vi "Process Image for Balls.vi"(0 "Src Image":T1, 1 "Color Mode 2":u16(ring)=2 items=["RGB", "HSL", "HSV", "HSI"], 5 "Image Dst":T1, 9 "Color":T3, 11 "Area Cutoff %":dbl=0.4) -> (4 "Src Image Out":T1, 8 "First Threshold":T1, 10 "Fitted":T1, 15 "Potential":T2(array[cluster]))   [LabVIEW 2015]
doc: "Search image for circular colored particles. A second pass extracts a portion of the image, widens the color range, and fits a circle to the edge of the result."
uses:
  <vilib>/vision/Image Controls.llb/IMAQ Image.ctl
  <vilib>/vision/NI_Vision_Development_Module.lvlib
panel:
  out "Particles":i32
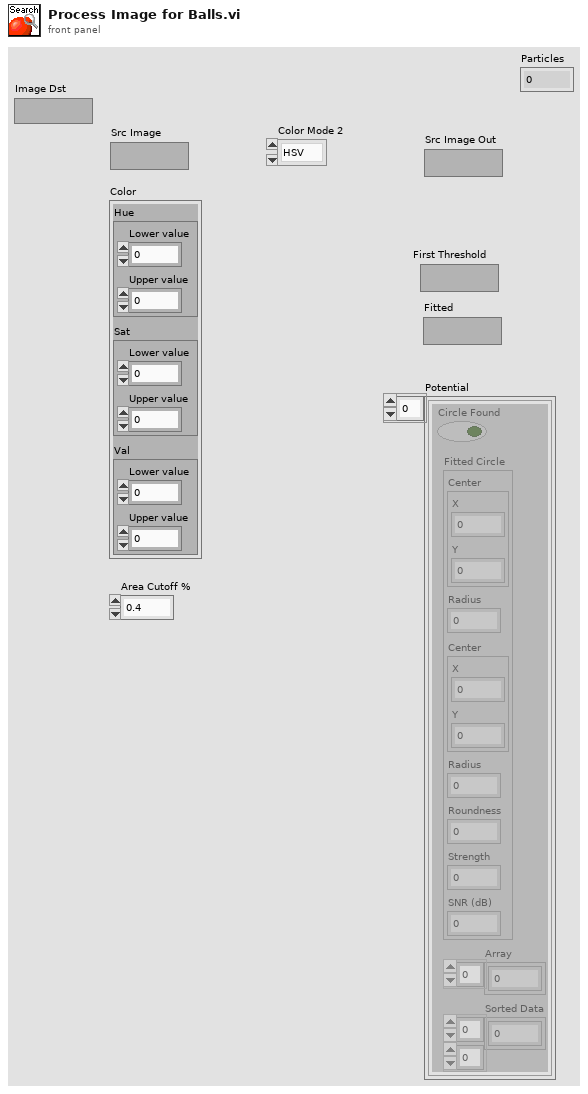
[diagram p1: front panel]
types:
  T1 = typedef "IMAQ Image.ctl" = refnum<image>
  T2 = cluster{"Circle Found":bool, "Fitted Circle":cluster{"Center":cluster{"X":sgl, "Y":sgl}, "Radius":dbl, "Center":cluster{"X":sgl, "Y":sgl}, "Radius":dbl, "Roundness":dbl, "Strength":dbl, "SNR (dB)":dbl}, "Array":dbl[], "Sorted Data":dbl[][]}[]
  T3 = cluster{"Hue ":cluster{"Lower value":i32, "Upper value":i32}, "Sat ":cluster{"Lower value":i32, "Upper value":i32}, "Val ":cluster{"Lower value":i32, "Upper value":i32}}
  T4 = typedef "Particle Parameters" = i32
  T5 = typedef "ROI Descriptor" = cluster{"Global Rectangle":i32[], "Contours":cluster{"ID":enum32{"External", "Internal"}, "Type":u32, "Coordinates":i32[]}[]}
  T6 = cluster{"Circle Found":bool, "Fitted Circle":cluster{"Center":cluster{"X":sgl, "Y":sgl}, "Radius":dbl, "Center":cluster{"X":sgl, "Y":sgl}, "Radius":dbl, "Roundness":dbl, "Strength":dbl, "SNR (dB)":dbl}, "Array":dbl[], "Sorted Data":dbl[][]}
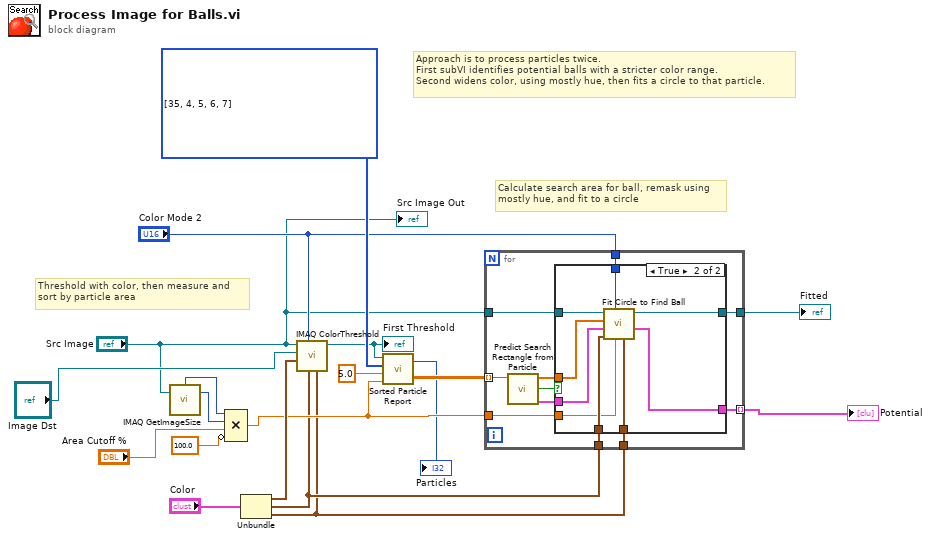
[diagram p0: block diagram]
diagram:
  w18 = T4[] [35, 4, 5, 6, 7] items=["Center of Mass X", "Center of Mass Y", "First Pixel X", "First Pixel Y", "Bounding Rect Left", "Bounding Rect Top", "Bounding Rect Right", "Bounding Rect Bottom", "Max Feret Diameter Start X", "Max Feret Diameter Start Y", "Max Feret Diameter End X", "Max Feret Diameter End Y", "Max Horiz. Segment Length Left", "Max Horiz. Segment Length Right", "Max Horiz. Segment Length Row", "-", "Bounding Rect Width", "Bounding Rect Height", "Bounding Rect Diagonal", "Perimeter", "Convex Hull Perimeter", "Holes' Perimeter", "Max Feret Diameter", "Equivalent Ellipse Major Axis", "Equivalent Ellipse Minor Axis", "Equivalent Ellipse Minor Axis (Feret)", "Equivalent Rect Long Side", "Equivalent Rect Short Side", "Equivalent Rect Diagonal", "Equivalent Rect Short Side (Feret)", "Average Horiz. Segment Length", "Average Vert. Segment Length", "Hydraulic Radius", "Waddel Disk Diameter", "-", "Area", "Holes' Area", "Particle & Holes' Area", "Convex Hull Area", "Image Area", "-", "Number of Holes", "Number of Horiz. Segments", "Number of Vert. Segments", "-", "Orientation", "Max Feret Diameter Orientation", "-", "% Area/Image Area", "% Area/(Particle & Holes' Area)", "Ratio of Equivalent Ellipse Axes", "Ratio of Equivalent Rect Sides", "-", "Elongation Factor", "Compactness Factor", "Heywood Circularity Factor", "Type Factor", "-", "Sum X", "Sum Y", "Sum XX", "Sum XY", "Sum YY", "Sum XXX", "Sum XXY", "Sum XYY", "Sum YYY", "-", "Moment of Inertia XX", "Moment of Inertia XY", "Moment of Inertia YY", "Moment of Inertia XXX", "Moment of Inertia XXY", "Moment of Inertia XYY", "Moment of Inertia YYY", "Norm. Moment of Inertia XX", "Norm. Moment of Inertia XY", "Norm. Moment of Inertia YY", "Norm. Moment of Inertia XXX", "Norm. Moment of Inertia XXY", "Norm. Moment of Inertia XYY", "Norm. Moment of Inertia YYY", "Hu Moment 1", "Hu Moment 2", "Hu Moment 3", "Hu Moment 4", "Hu Moment 5", "Hu Moment 6", "Hu Moment 7"] ("Pixel Measurements")
  # "Approach is to process particles twice.\nFirst subVI identifies potential balls with a stricter color range.\nSecond widens color, using mostly hue, then fits a circle to that particle."
  # "Threshold with color, then measure and\nsort by particle area"
  # "Calculate search area for ball, remask using\nmostly hue, and fit to a circle"
  n1 = call "IMAQ GetImageSize"("Image"="Src Image") -> ("Y Resolution"=w9:i32, "X Resolution"=w10:i32)  [unwired: 3 in, 1 out]
  n2 = Compound Arithmetic op=MULTIPLY(w10, w9, "Area Cutoff %", invert 100.0 ("value")) -> (w7:dbl)
  n3 = Unbundle("Color") -> ("Hue"=w16:cluster{"Lower value":i32, "Upper value":i32}, "Sat"=w2:cluster{"Lower value":i32, "Upper value":i32}, "Val"=w1:cluster{"Lower value":i32, "Upper value":i32})
  n4 = call "IMAQ ColorThreshold"("Blue or Luma or Val or Inten Range"=w1, "Green or Sat Range"=w2, "Color Mode"="Color Mode 2", "Red or Hue Range"=w16, "Image Dst"="Image Dst", "Image Src"="Src Image") -> ("Image Dst Out"=w15:T1)  [unwired: 4 in, 1 out]
  "First Threshold" <- w15
  n5 = call "Sorted Particle Report.vi"("Area Size Limit"=w7, "Particle Count Limit"=5.0, "Pixel Measurements"=w18, "Image in"=w15) -> ("Sorted Data"=w14:dbl[][], "Particles"=→"Particles":i32)
  n6 = for {
    tunnel: w14 -> [w30] mode=indexing
    tunnel: [w28] -> w12 mode=indexing
    tunnel: w2 -> [w26]
    tunnel: w7 -> [w23]
    tunnel: "Color Mode 2" -> [w24]
    tunnel: "Src Image" -> [w22]
    tunnel: [w21] -> w19
    tunnel: w1 -> [w20]
    n7 = call "Predict Search Rectangle from Particle.vi"("Sorted Data"=w30) -> ("ROI Descriptor"=w25:T5, "Valid"=w27:bool, "Rectangle ltrb"=w29:dbl[])  [unwired: 8 in]
    n8 = case shown="True" w27 {
      tunnel: w29 -> [_ w36]
      tunnel: [_ w40] -> w28
      tunnel: w22 -> [w31 w35]
      tunnel: w26 -> [_ w37]
      tunnel: w25 -> [_ w39]
      tunnel: w24 -> [_ w38]
      tunnel: w23 -> [_ w34]
      tunnel: [w31 w33] -> w21
      tunnel: w20 -> [_ w32]
      frame False {
      }
      frame True {
        n9 = call "Fit Circle to Find Ball.vi"("Val"=w32, "Area Size Limit"=w34, "Color Mode"=w38, "Sat"=w37, "ROI Descriptor"=w39, "Rectangle ltrb"=w36, "Color Image In"=w35) -> ("Potential Ball"=w40:T6, "Image out"=w33:T1)  [unwired: 3 in]
      }
    }
  }
  "Fitted" <- w19
  "Potential" <- w12
  "Src Image Out" <- "Src Image"
